vi "V1_DAQ_config.vi"() -> (1 "error out":errorcluster, 2 "task out":refnum<k21>)   [LabVIEW 2020]
uses:
  <vilib>/DAQmx/create/channels.llb/DAQmx Create Channel (AI-Voltage-Basic).vi
  <vilib>/DAQmx/configure/timing.llb/DAQmx Timing (Sample Clock).vi
panel:
  in  "input terminal configuration":i32(ring)=-1 items=["Default"=-1, "RSE"=10083, "NRSE"=10078, "Differential"=10106, "Pseudodifferential"=12529]
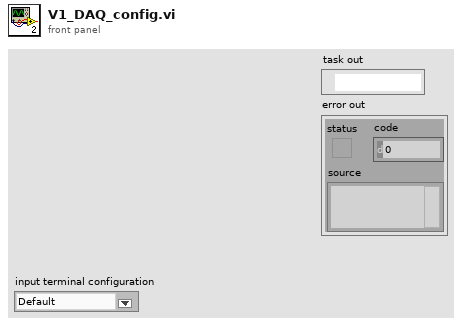
[diagram p1: front panel]
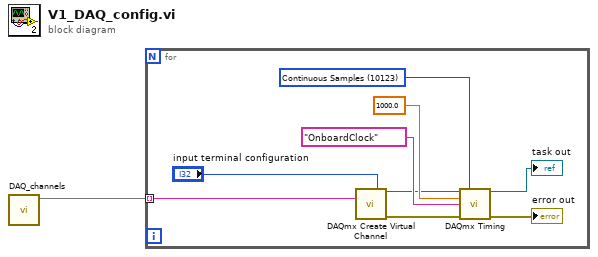
[diagram p0: block diagram]
diagram:
  n1 = call "DAQ_channels.vi"() -> (3:w1)  [unwired: 9 in, 2 out]
  n2 = for {
    tunnel: w1 -> [w2] mode=indexing
    w10 = 10123 items=["Finite Samples"=10178, "Continuous Samples"=10123, "Hardware Timed Single Point"=12522] ("sample mode")
    n3 = call-poly <vilib>:"DAQmx Create Virtual Channel.vi"("input terminal configuration"="input terminal configuration", "physical channels"=w2) -> ("task out"=w5:refnum<k21>, "error out"=w6:errorcluster)  [unwired: 12 in]
    n4 = call-poly <vilib>:"DAQmx Timing.vi"("task/channels in"=w5, "sample mode"=w10, "rate"=1000.0 ("sample rate"), "source"=tag "OnboardClock", "error in"=w6) -> ("task out"=→"task out":refnum<k21>, "error out"=→"error out":errorcluster)  [unwired: 9 in]
  }
